vi "fbp-worker.vi"(6 "pixels for projections":refnum<queue>, 7 "keep pixels?":bool, 8 "Centre":i32[](array[numeric]), 9 "Write queue":refnum<queue>, 10 "Image Properties":T1, 11 "Work queue in":refnum<queue>) -> (1 "New Angle":dbl, 2 "progress angle":dbl, 3 "results":sgl[](array[numeric]))   [LabVIEW 2013]
uses:
  tags_cluster.ctl
  imagereconstruction/x64/Debug/labviewdll.dll
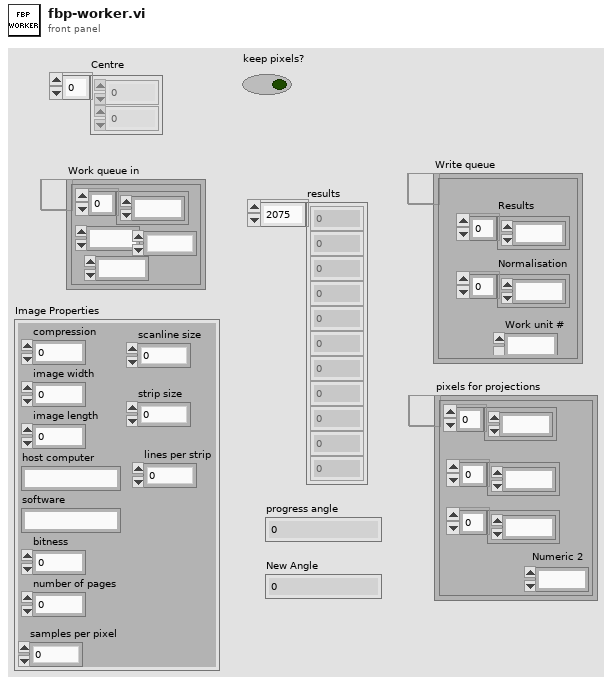
[diagram p1: front panel]
types:
  T1 = typedef "tags_cluster.ctl" = cluster{"compression":i32, "image width":i32, "image length":i32, "host computer":string, "software":string, "bitness":i32, "number of pages":i32, "samples per pixel":i32, "scanline size":i32, "strip size":i32, "lines per strip":i32}
  T2 = cluster{u8[], dbl, "Numeric":i32, "Numeric 2":i32}
  T3 = cluster{"normalisation":i32[], "pixels":i32[], "count":i32[], "Numeric 2":i32}
  T4 = cluster{"results":sgl[], "normalisation":i32[], "Numeric":i32}
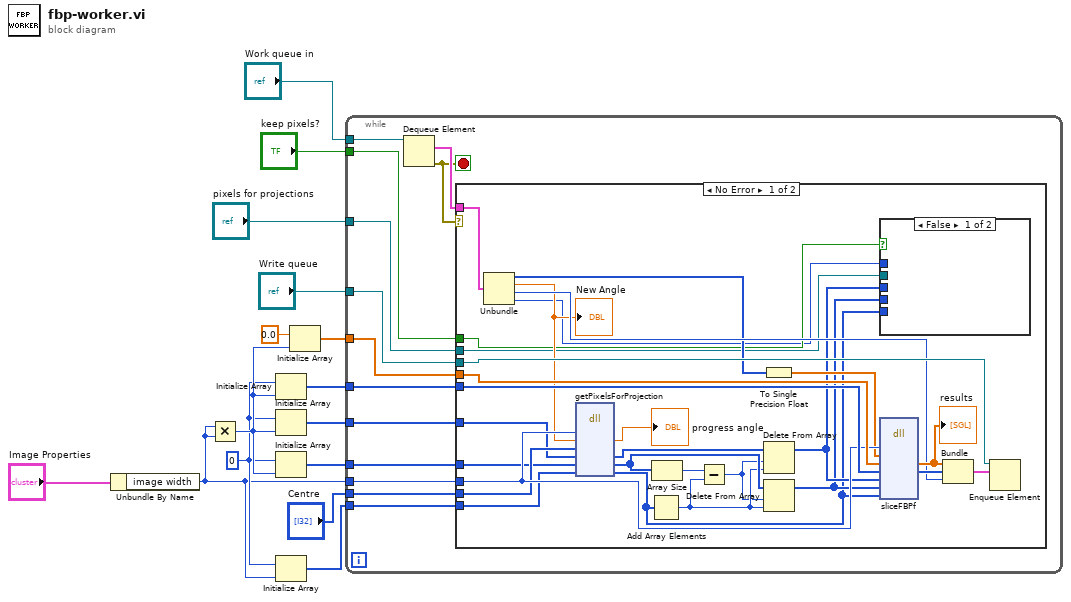
[diagram p0: block diagram]
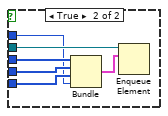
[diagram p2: hidden frame]
diagram:
  w4 = 0 ("element")
  n1 = Unbundle By Name("Image Properties") -> ("image width"=w3:i32)
  n2 = Multiply(x=w3, y=w3) -> (x*y=w8:i32)
  n3 = Initialize Array(w4, w8) -> (w13:i32[])
  n4 = Initialize Array(w4, w8) -> (w7:i32[])
  n5 = Initialize Array(w4, w8) -> (w6:i32[])
  n6 = Initialize Array(w4, w3) -> (w2:i32[])
  n7 = Initialize Array(sgl 0.0 ("element"), w8) -> (w15:sgl[])
  n8 = while {
    tunnel: "Work queue in" -> [w28]
    tunnel: w3 -> [w27]
    tunnel: w13 -> [w26]
    tunnel: w15 -> [w25]
    tunnel: "Write queue" -> [w22]
    tunnel: "Centre" -> [w21]
    tunnel: w7 -> [w20]
    tunnel: w6 -> [w19]
    tunnel: "pixels for projections" -> [w18]
    tunnel: w2 -> [w17]
    tunnel: "keep pixels?" -> [w16]
    stop <- w23 stop-if-true
    n9 = Dequeue Element(queue=w28) -> (element=w24:T2, error out=w23:errorcluster)  [unwired: 2 in, 2 out]
    n10 = case shown="No Error" w23 {
      tunnel: w27 -> [w48 _]
      tunnel: w26 -> [w56 _]
      tunnel: w25 -> [w55 _]
      tunnel: w24 -> [w54 _]
      tunnel: w22 -> [w53 _]
      tunnel: w21 -> [w47 _]
      tunnel: w20 -> [w45 _]
      tunnel: w19 -> [w44 _]
      tunnel: w18 -> [w34 _]
      tunnel: w17 -> [w37 _]
      tunnel: w16 -> [w33 _]
      frame No Error {
        n11 = Unbundle(w54) -> (w36:u8[], w43:dbl, "Numeric"=w49:i32, "Numeric 2"=w29:i32)
        "New Angle" <- w43
        n12 = dll-call lib="D:/work/uni/FYP/reconrepo/imagereconstruction/x64/Debug/labviewdll.dll" fn="getPixelsForProjection"("w"=w48, "angle"=w43, "centre"=w47, "normalisation"=w45, "pixels"=w44, "count"=w37) -> ("angle"=→"progress angle":dbl, "normalisation"=w38:i32[], "pixels"=w42:i32[], "count"=w30:i32[])  [unwired: 6 in, 2 out]
        n13 = Add Array Elements(numeric array=w30) -> (sum=w40:i32)
        n14 = Array Size(array=w42) -> (size(s)=w41:i32)
        n15 = Subtract(x=w41, y=w40) -> (x-y=w39:i32)
        n16 = To Single Precision Float(number=w36) -> (single precision float=w35:sgl[])
        n17 = Delete From Array(array=w38, length=w39, index=w40) -> (array with subset deleted=w32:i32[])  [unwired: 1 out]
        n18 = Delete From Array(array=w42, length=w39, index=w40) -> (array with subset deleted=w31:i32[])  [unwired: 1 out]
        n19 = case shown="False" w33 {
          tunnel: w34 -> [_ w62]
          tunnel: w32 -> [_ w60]
          tunnel: w31 -> [_ w59]
          tunnel: w30 -> [_ w58]
          tunnel: w29 -> [_ w57]
          frame False {
          }
          frame True {
            n20 = Bundle("normalisation"=w60, "pixels"=w59, "count"=w58, "Numeric 2"=w57) -> (w61:T3)  [unwired: 1 in]
            n21 = Enqueue Element(queue=w62, element=w61) -> ()  [unwired: 2 in, 3 out]
          }
        }
        n22 = dll-call lib="D:/work/uni/FYP/reconrepo/imagereconstruction/x64/Debug/labviewdll.dll" fn="sliceFBPf"("w"=w48, "strip"=w35, "results"=w55, "normalisation"=w56, "rayNormalisation"=w32, "pixels"=w31, "count"=w30) -> ("results"=w51:sgl[], "normalisation"=w50:i32[])  [unwired: 9 in, 2 out]
        "results" <- w51
        n23 = Bundle("results"=w51, "normalisation"=w50, "Numeric"=w49) -> (w52:T4)  [unwired: 1 in]
        n24 = Enqueue Element(queue=w53, element=w52) -> ()  [unwired: 2 in, 3 out]
      }
      frame Error {
      }
    }
  }
